vi "Joints_Filter.vi"(10 "Modelo":dbl[][](array[numeric]), 11 "Kinect 1":dbl[][](array[numeric])) -> (2 "Array Válido":dbl[][](array[numeric]), 3 "Joints":dbl[](array[numeric]))   [LabVIEW 2016]
panel:
  out "Nível de Confiança":dbl[](array[numeric])
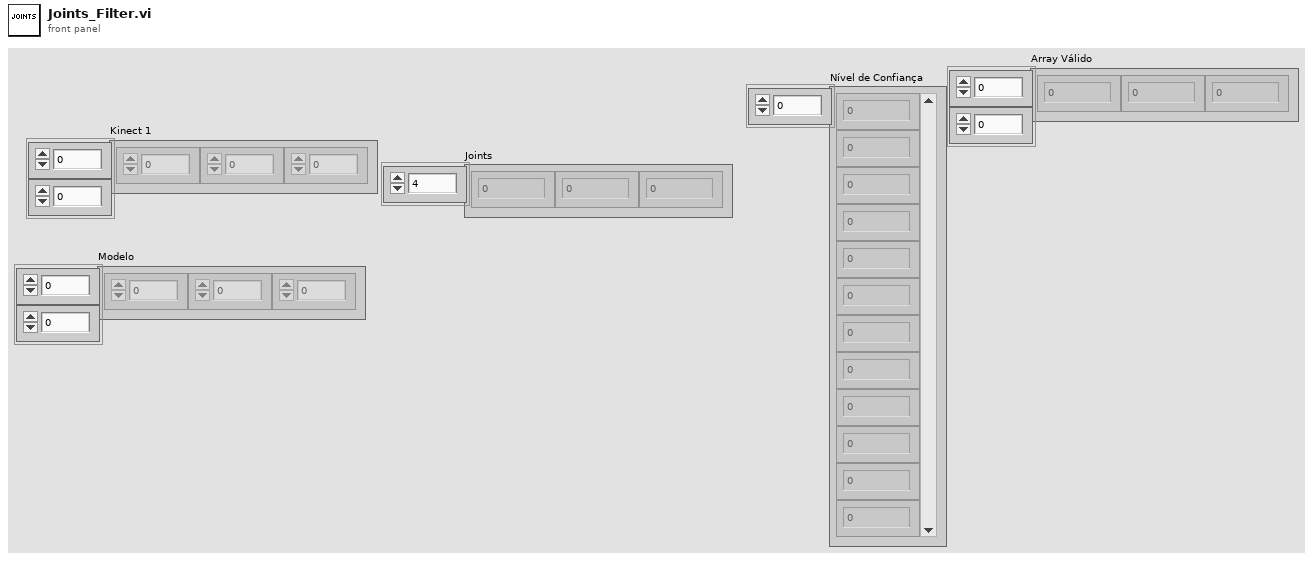
[diagram p1: front panel]
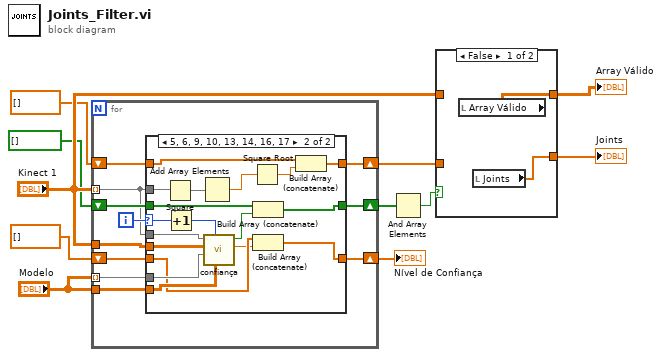
[diagram p0: block diagram]
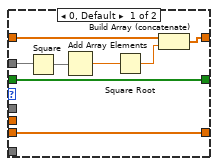
[diagram p3: hidden frame]
diagram:
  n1 = for {
    tunnel: "Kinect 1" -> [w14] mode=indexing
    tunnel: "Modelo" -> [w20] mode=indexing
    tunnel: "Kinect 1" -> [w19]
    tunnel: "Modelo" -> [w21]
    shift-right: [w18] -> w6
    shift-left: dbl[] [] -> [w17]
    shift-right: [w16] -> w9
    shift-left: bool[] [] -> [w15]
    shift-right: [w13] -> w7
    shift-left: dbl[] [] -> [w12]
    i -> [w22]
    n2 = case shown="5, 6, 9, 10, 13, 14, 16, 17" w22 {
      selector: w22 -> [_ w44]
      tunnel: w14 -> [_ w48]
      tunnel: w21 -> [_ w47]
      tunnel: w20 -> [_ w46]
      tunnel: w19 -> [_ w45]
      tunnel: [w30 w40] -> w18
      tunnel: w17 -> [w30 w42]
      tunnel: [w29 w38] -> w16
      tunnel: w15 -> [w29 w37]
      tunnel: w14 -> [w27 w34]
      tunnel: [w24 w32] -> w13
      tunnel: w12 -> [w23 w31]
      frame 0, Default {
        n3 = Square(x=w27) -> (x^2=w26:dbl[])
        n4 = Add Array Elements(numeric array=w26) -> (sum=w28:dbl)
        n5 = Square Root(x=w28) -> (sqrt(x)=w25:dbl)
        n6 = Build Array (concatenate)(w23, w25) -> (w24:dbl[])
      }
      frame 5, 6, 9, 10, 13, 14, 16, 17 {
        n7 = Square(x=w34) -> (x^2=w35:dbl[])
        n8 = Increment(x=w44) -> (x+1=w43:i32)
        n9 = Add Array Elements(numeric array=w35) -> (sum=w36:dbl)
        n10 = call "confiança.vi"("Modelo in"=w47, "Numeric Control in"=w43, "Modelo"=w46, "Kinect in"=w45, "Kinect 1"=w48) -> ("Numeric Control out"=w41:dbl, "Confiável"=w39:bool)  [unwired: 5 in]
        n11 = Square Root(x=w36) -> (sqrt(x)=w33:dbl)
        n12 = Build Array (concatenate)(w37, w39) -> (w38:bool[])
        n13 = Build Array (concatenate)(w42, w41) -> (w40:dbl[])
        n14 = Build Array (concatenate)(w31, w33) -> (w32:dbl[])
      }
    }
  }
  "Nível de Confiança" <- w6
  n15 = And Array Elements(Boolean array=w9) -> (logical AND=w8:bool)
  n16 = case shown="False" w8 {
    tunnel: w7 -> [_ w51]
    tunnel: "Kinect 1" -> [_ w52]
    tunnel: [w50 w52] -> w2
    tunnel: [w49 w51] -> w1
    frame False {
      n17 = local read "Array Válido"() -> (w50:dbl[][])
      n18 = local read "Joints"() -> (w49:dbl[])
    }
    frame True {
    }
  }
  "Joints" <- w1
  "Array Válido" <- w2
